vi "CCM provide total length.vi"(8 "error in":errorcluster, 10 "total length":i32, 11 "lvlibcrypto digest in":refnum<class "lvlibcrypto cipher.lvclass">) -> (0 "error out":errorcluster, 3 "lvlibcrypto digest out":refnum<class "lvlibcrypto cipher.lvclass">)   [LabVIEW 2016, in "lvlibcrypto cipher.lvclass"]
uses:
  lvlibcrypto cipher.lvclass
  lvlibcrypto cipher.lvclass/lvlibcrypto cipher.ctl
  lv tls dll.lvlib
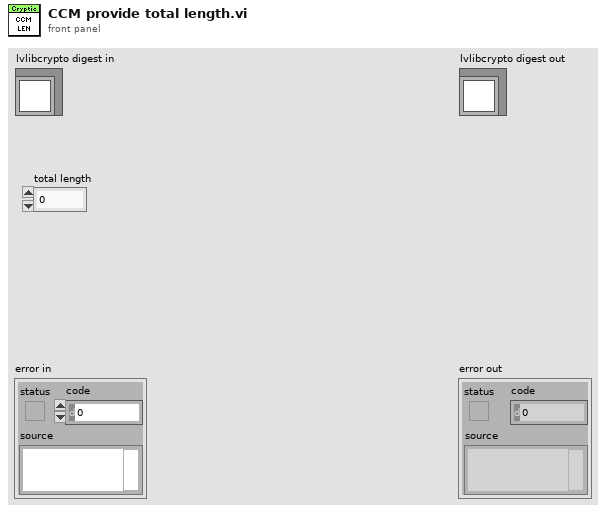
[diagram p1: front panel]
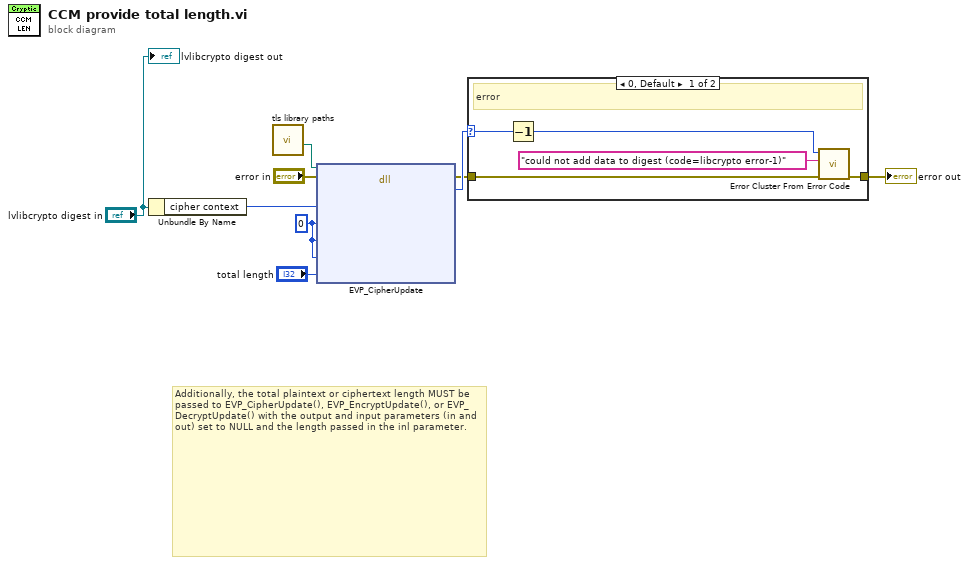
[diagram p0: block diagram]
diagram:
  w1 = u64 0 ("out")
  # "Additionally, the total plaintext or ciphertext length MUST be passed to EVP_CipherUpdate(), EVP_EncryptUpdate(), or EVP_DecryptUpdate() with the output and input parameters (in and out) set to NULL and the length passed in the inl parameter."
  n1 = Unbundle By Name("lvlibcrypto digest in") -> ("cipher context"=w3:u64)
  n2 = call "tls library paths.vi"() -> ("libcrypto"=w8:path)  [unwired: 8 in, 3 out]
  n3 = dll-call lib="C:/Users/IEUser/Desktop/tlssimple/libcrypto-41.dll" fn="EVP_CipherUpdate"(path in=w8, error in="error in", "context"=w3, "out"=w1, "outlength"=w1, "in"=w1, "inlength"="total length") -> (error out=w4:errorcluster, "ret"=w5:i32)  [unwired: 6 in, 1 out]
  n4 = case shown="0, Default" w5 {
    selector: w5 -> [w12 _]
    tunnel: [w13 w15] -> w7
    tunnel: w4 -> [w14 w15]
    frame 0, Default {
      # "error"
      n5 = Decrement(x=w12) -> (x-1=w11:i32)
      n6 = call <vilib>:"Error Cluster From Error Code.vi"("error in (no error)"=w14, "error message (\"\")"="could not add data to digest (code=libcrypto error-1)" ("error message (\"\")"), "error code (0)"=w11) -> ("error out"=w13:errorcluster)  [unwired: 6 in]
    }
    frame 1 {
      # "success"
    }
  }
  "error out" <- w7
  "lvlibcrypto digest out" <- "lvlibcrypto digest in"
